vi "zi_S1_S2_DAQ2.vi"() -> ()   [LabVIEW 2021]
uses:
  <instrlib>/Zurich Instruments LabOne/Zurich Instruments LabOne.lvlib
panel:
  in  "zi Address":string
  out "Waveform Chart":dbl(graph)
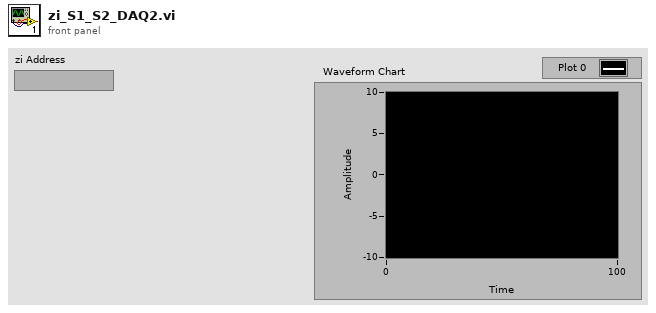
[diagram p1: front panel]
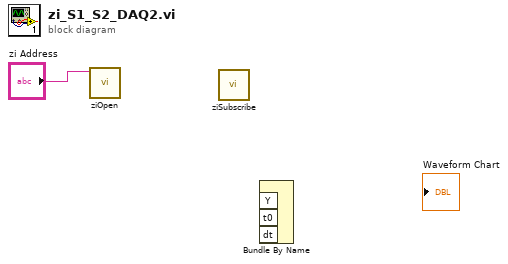
[diagram p0: block diagram]
diagram:
  n1 = call <instrlib>:"ziOpen.vi"("Address"="zi Address") -> ()  [unwired: 3 in, 3 out]
  n2 = call <instrlib>:"ziSubscribe.vi"() -> ()  [unwired: 4 in, 2 out]
  n3 = Bundle By Name() -> ()  [unwired: 4 in, 1 out]
